vi "Ramp Voltage.vi"(6 "Step":dbl=1.0 format="%#_13g", 7 "channel list":string="WL_SEL, BL_EN, WL_EN", 8 "error in (no error)":errorcluster, 9 "Final Value":dbl=5.0 format="%#_13g", 10 "Initial Value":dbl, 11 "instrument handle":refnum<k15>) -> (0 "error out":errorcluster, 3 "instrument handle out":refnum<k15>)   [LabVIEW 2018]
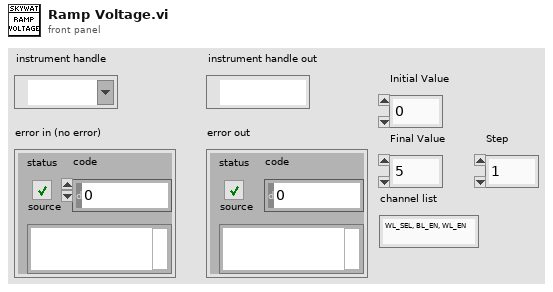
[diagram p1: front panel]
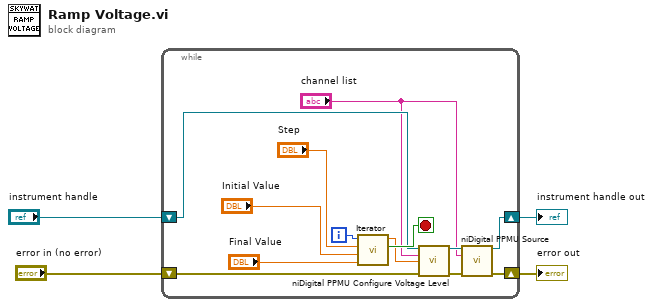
[diagram p0: block diagram]
diagram:
  n1 = while {
    shift-right: [w8] -> w3
    shift-left: "instrument handle" -> [w10]
    shift-right: [w7] -> w4
    shift-left: "error in (no error)" -> [w9]
    i -> [w15]
    stop <- w13 stop-if-true
    n2 = call "Iterator.vi"("Final Value"="Final Value", "Initial Value"="Initial Value", "Step"="Step", "i"=w15) -> ("End Loop"=w13:bool, "Current Value"=w11:dbl)  [unwired: 6 in]
    n3 = call <instrlib>:"niDigital PPMU Configure Voltage Level.vi"("instrument handle"=w10, "channel list"="channel list", "voltage level (V)"=w11, "error in"=w9) -> ("instrument handle out"=w16:refnum<k15>, "error out"=w17:errorcluster)  [unwired: 10 in]
    n4 = call <instrlib>:"niDigital PPMU Source.vi"("instrument handle"=w16, "channel list"="channel list", "error in"=w17) -> ("instrument handle out"=w8:refnum<k15>, "error out"=w7:errorcluster)  [unwired: 11 in]
  }
  "error out" <- w4
  "instrument handle out" <- w3
